vi "PH_Beckhoff_Watchdog.panel.vi"(0 "object ref":refnum<vi>, 5 "error in (no error)":errorcluster) -> (19 "error out":errorcluster)   [LabVIEW 2014, in "PH_Beckhoff_Watchdog.lvlib"]
doc: "By this VI a hardware switch can be monitored and switched. \n\nThe indicators \"FALSE\", \"TRUE\" and \"SWITCH STATE\" show the value of the Beckhoff-Tag: blue indicates bad tag status reference problems, darkgreen false and lightgreen true. If everything is working fine, \"FALSE\" and \"SWITCH STATE\" should show the same value, while \"TRUE\" has the opposite value. The caption of the sensors for \"FALSE\" and \"TRUE\" are taken out of the database. In case of only one or no sensor these GUI elements are not shown at all.\n\nThe oval button switches. It should be in the same state as the \"SWITCH STATE\" indicator. \n\n\"Delete Instance\" disconnects and removes the instance from the PCS.\n\n\nLicense Agreement for this software:\n\nCopyright (C)\nGesellschaft für Schwerionenforschung, GSI\nPlanckstr. 1\n64291 Darmstadt\nGermany\n\nContact: D.Beck@gsi.de \n\nThis program is free software; you can redistribute it and/or modify it under the terms of the GNU General Public License as published by the Free Software Foundation; either version 2 of the license, or (at your option) any later version.\n\nThis program is distributed in the hope that it will be useful, but WITHOUT ANYW ARRANTY; without even the implied warranty of MERCHANTABILITY or FITNESS FOR A PARTICULAR PURPOSE. See the GNU General License for more details (http://www.gnu.org).\n\nGesellschaft für Schwerionenforschung, GSI\nPlanckstr. 1, 64291 Darmstadt, Germany\nFor all questions and ideas contact: M.Richter@gsi.de, H.Brand@gsi.de or D.Beck@gsi.de.\nLast update: 18-DEC-2002"
uses:
  PH_Beckhoff_Watchdog.lvlib
  PH_Basics/PH_StatusHandler/PH_StatusHandler.GUI element.ctl
  PH_Basics/PH_StatusHandler/PH_StatusHandler.Status.ctl
  CS_Core/CSObj/CSObj.lvlib
  PH_Basics/PH_Common/PH_Common.lvlib
  PH_Basics/PH_Class/PH_Class.lvlib
  PH_Basics/PH_StatusHandler/PH_StatusHandler.lvlib
panel:
  out "MA_Beckhoff_StepMot_DC_ok":u32(colorbox) caption="z6beck006"
  out "Exp_LL_Beckhoff-16BB_DC_int_ok":u32(colorbox) caption="phbeckrack009"
  out "COS_Beckhoff-16BB_DC_int_ok":u32(colorbox) caption="phbeckrack004"
  in  "Exit":bool
  out "Status":T1 caption="Enabling State"
  out "Timing_DC_ok":u32(colorbox)=6618880 caption="phbeckrack024"
  out "MA-Rack4-Beckhoff-PU_DC_ok":u32(colorbox)=6618880 caption="phbeckrack021"
  out "MA-Rack3-Beckhoff-PU_DC_ok":u32(colorbox)=6618880 caption="phbeckrack020"
  out "MA-Rack2-Beckhoff-PU_DC_ok":u32(colorbox)=6618880 caption="phbeckrack019"
  out "MA-Rack1-Beckhoff-PU_DC_ok":u32(colorbox)=6618880 caption="phbeckrack018"
  out "PP_Control_DC_ok":u32(colorbox)=6618880 caption="phbeckrack014"
  out "PA-45mm-Beckhoff-PU_DC_ok":u32(colorbox)=6618880 caption="phbeckrack025"
  out "PA-19mm-Beckhoff-PU_DC_ok":u32(colorbox)=6618880 caption="phbeckrack012"
  out "PPMA_Beckhoff-Dumprods_DC_ok":u32(colorbox)=6618880 caption="phbeckrack017"
  out "PIL_DC_ok8":u32(colorbox)=6618880 caption="phbeckrack023"
  out "PIL_DC_ok1":u32(colorbox)=6618880 caption="phbeckrack022"
  out "Exp_LB_Beckhoff-10BB-Plus_DC_int_ok":u32(colorbox) caption="phbeckrack015"
  out "MA_Beckhoff-10BB-Plus_DC_ext_ok":u32(colorbox) caption="phbeckrack008"
  out "MAS_Beckhoff-16BB_DC_int_ok":u32(colorbox) caption="phbeckrack005"
  out "PA_Beckhoff-16BB_DC_int_ok":u32(colorbox) caption="phbeckrack007"
  out "MA01_DC_ok":u32(colorbox) caption="phbeckrack011"
  out "Z6_ST_Beckhoff-16BB_DC_int_ok":u32(colorbox) caption="phbeckrack001"
  in  "Delete":bool
  # "PCS"
  # "3.40"
  # "Beam Diag.\nPLH 2.002"
  # "ELT  PLH 2.004"
  # "Laser Labor\nPLH 1.001"
  # "Test Labor\nPLH 2.001"
  # "Stairway"
  # "Stairway"
  # "Laser Bay\nPLH 1.002"
  # "PKR\nPLH 2.007"
  # "HV Room\nPLH 2.005"
  # "Exp 4: Z6"
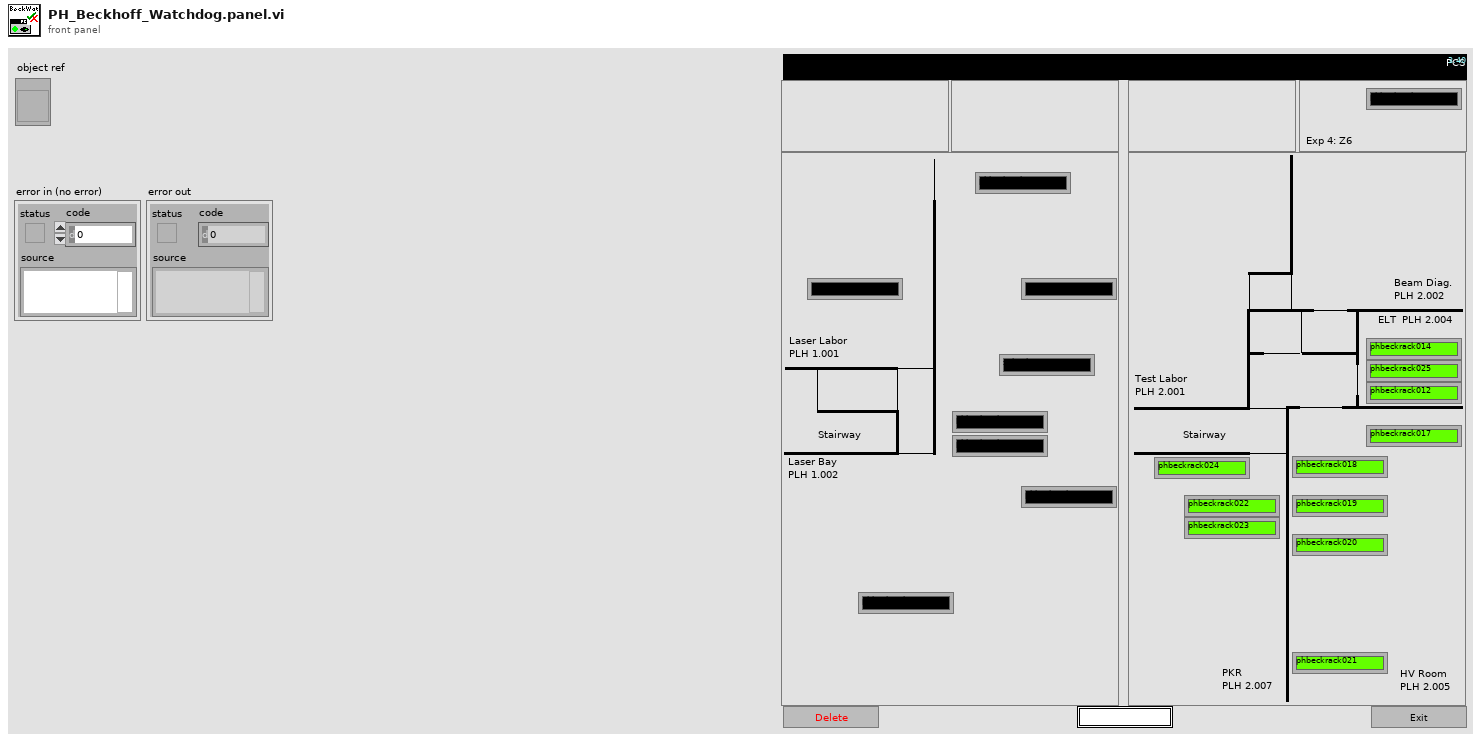
[diagram p1: front panel]
types:
  T1 = typedef "PH_StatusHandler.lvlib/PH_StatusHandler.GUI element.ctl" = u16
  T2 = typedef "PH_StatusHandler.lvlib/PH_StatusHandler.Status.ctl" = i16
  T3 = typedef "PH_Beckhoff_Watchdog.lvlib/PH_Beckhoff_Watchdog.i attribute.ctl" = cluster{"Info":cluster{"GUI Ref":refnum<vi>, "Status":T2}[]}
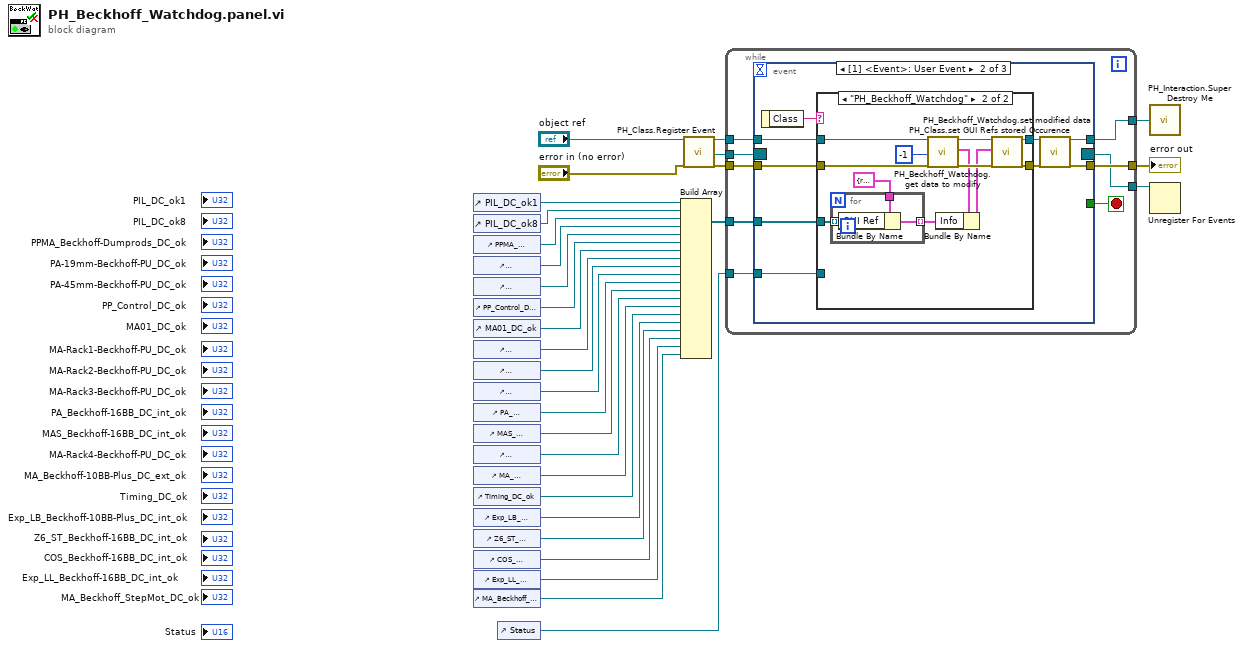
[diagram p0: block diagram]
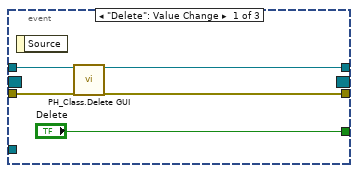
[diagram p2: hidden frame]
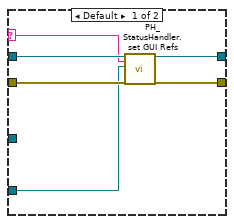
[diagram p3: hidden frame]
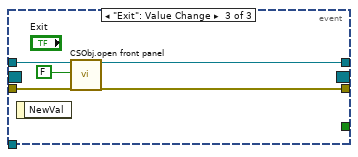
[diagram p4: hidden frame]
diagram:
  n1 = control-ref of="PIL_DC_ok1"() -> (w13:refnum<vi>)
  n2 = control-ref of="PIL_DC_ok8"() -> (w14:refnum<vi>)
  n3 = control-ref of="PPMA_Beckhoff-Dumprods_DC_ok"() -> (w15:refnum<vi>)
  n4 = control-ref of="PA-19mm-Beckhoff-PU_DC_ok"() -> (w29:refnum<vi>)
  n5 = control-ref of="PA-45mm-Beckhoff-PU_DC_ok"() -> (w28:refnum<vi>)
  n6 = control-ref of="PP_Control_DC_ok"() -> (w27:refnum<vi>)
  n7 = control-ref of="MA01_DC_ok"() -> (w26:refnum<vi>)
  n8 = control-ref of="MA-Rack1-Beckhoff-PU_DC_ok"() -> (w25:refnum<vi>)
  n9 = control-ref of="MA-Rack2-Beckhoff-PU_DC_ok"() -> (w24:refnum<vi>)
  n10 = control-ref of="MA-Rack3-Beckhoff-PU_DC_ok"() -> (w23:refnum<vi>)
  n11 = control-ref of="PA_Beckhoff-16BB_DC_int_ok"() -> (w22:refnum<vi>)
  n12 = control-ref of="MAS_Beckhoff-16BB_DC_int_ok"() -> (w21:refnum<vi>)
  n13 = control-ref of="MA-Rack4-Beckhoff-PU_DC_ok"() -> (w20:refnum<vi>)
  n14 = control-ref of="MA_Beckhoff-10BB-Plus_DC_ext_ok"() -> (w19:refnum<vi>)
  n15 = control-ref of="Timing_DC_ok"() -> (w18:refnum<vi>)
  n16 = control-ref of="Exp_LB_Beckhoff-10BB-Plus_DC_int_ok"() -> (w17:refnum<vi>)
  n17 = control-ref of="Z6_ST_Beckhoff-16BB_DC_int_ok"() -> (w12:refnum<vi>)
  n18 = control-ref of="COS_Beckhoff-16BB_DC_int_ok"() -> (w11:refnum<vi>)
  n19 = control-ref of="Exp_LL_Beckhoff-16BB_DC_int_ok"() -> (w10:refnum<vi>)
  n20 = control-ref of="MA_Beckhoff_StepMot_DC_ok"() -> (w2:refnum<vi>)
  n21 = control-ref of="Status"() -> (w1:refnum<vi>)
  n22 = Build Array(w13, w14, w15, w29, w28, w27, w26, w25, w24, w23, w22, w21, w20, w19, w18, w17, w12, w11, w10, w2) -> (w5:refnum<vi>[])
  n23 = call "PH_Class.Register Event.vi"("i ref in"="object ref", "error in (no error)"="error in (no error)") -> ("i ref out"=w9:refnum<vi>, "Event Registration Refnum"=w7:refnum<event-registration>, "error out"=w8:errorcluster)  [unwired: 15 in]
  n24 = while {
    tunnel: w9 -> [w36]
    tunnel: [w35] -> w16
    tunnel: w8 -> [w38]
    tunnel: [w37] -> w30
    tunnel: w7 -> [w34]
    tunnel: [w33] -> w6
    tunnel: w5 -> [w32]
    tunnel: w1 -> [w31]
    stop <- w39 stop-if-true
    n25 = event shown="[1] <Event>: User Event" {
      selector: w34 -> [_ _ _]
      dyn-events: [_ _ _] -> w33
      timeout: _ -> [_ _ _]
      tunnel: ["Delete" _ _] -> w39
      tunnel: w36 -> [w43 w51 w78]
      tunnel: w38 -> [w42 w49 w76]
      tunnel: [w41 w52 w75] -> w37
      tunnel: [w40 w53 w77] -> w35
      tunnel: w32 -> [_ w47 _]
      tunnel: w31 -> [_ w46 _]
      event "Delete": Value Change {
        n26 = event-data() -> ()  [unwired: 1 in, 1 out]
        n27 = call "PH_Class.Delete GUI.vi"("VI in"=w43, "error in (no error)"=w42) -> ("VI out"=w40:refnum<vi>, "error out"=w41:errorcluster)  [unwired: 16 in]
      }
      event User Event {
        n28 = event-data() -> ("Class"=w45:string)  [unwired: 1 in]
        n29 = case shown="\"PH_Beckhoff_Watchdog\"" w45 {
          selector: w45 -> [w55 _]
          tunnel: w51 -> [w57 w65]
          tunnel: [w56 w64] -> w50
          tunnel: w49 -> [w59 w63]
          tunnel: [w58 w62] -> w48
          tunnel: w47 -> [_ w61]
          tunnel: w46 -> [w54 _]
          frame Default {
            n30 = call "PH_StatusHandler.set GUI Refs.vi"("i ref in"=w57, "Class"=w55, "GUI Ref"=w54, "error in (no error)"=w59) -> ("i ref out"=w56:refnum<vi>, "error out"=w58:errorcluster)  [unwired: 14 in]
          }
          frame "PH_Beckhoff_Watchdog" {
            n31 = for {
              tunnel: cluster{"GUI Ref":refnum<vi>, "Status":T2} {"GUI Ref"=refnum, "Status"=0} ("Cluster") -> [w74]
              tunnel: [w73] -> w66 mode=indexing
              tunnel: w61 -> [w72] mode=indexing
              n32 = Bundle By Name(cluster=w74, "GUI Ref"=w72) -> (w73:cluster{"GUI Ref":refnum<vi>, "Status":T2})
            }
            n33 = call "PH_Beckhoff_Watchdog.get data to modify.vi"("i ref in"=w65, "ms timeout (10000)"=-1, "error in (no error)"=w63) -> ("i ref out"=w71:refnum<vi>, "i attribute"=w68:T3, "error out"=w70:errorcluster)  [unwired: 13 in, 1 out]
            n34 = Bundle By Name(cluster=w68, "Info"=w66) -> (w67:T3)
            n35 = call "PH_Beckhoff_Watchdog.set modified data.vi"("i ref in"=w71, "i attribute"=w67, "error in (no error)"=w70) -> ("i ref out"=w64:refnum<vi>, "error out"=w62:errorcluster)  [unwired: 15 in]
          }
        }
        n36 = call "PH_Class.set GUI Refs stored Occurence.vi"("i ref in"=w50, "error in (no error)"=w48) -> ("i ref out"=w53:refnum<vi>, "error out"=w52:errorcluster)  [unwired: 16 in]
      }
      event "Exit": Value Change {
        n37 = event-data() -> ()  [unwired: 1 in, 1 out]
        n38 = call "CSObj.open front panel.vi"("i ref in"=w78, "frontPanelOpen"=FALSE ("front panel open"), "error in (no error)"=w76) -> ("i ref out"=w77:refnum<vi>, "error out"=w75:errorcluster)  [unwired: 15 in]
      }
    }
  }
  "error out" <- w30
  n39 = call "PH_Interaction.Super Destroy Me.vi"("i ref out"=w16) -> ()
  n40 = Unregister For Events(event registration refnum=w6) -> ()  [unwired: 1 in, 1 out]
